vi "Global - UI Stream and Variable Connections.vi"() -> ()   [LabVIEW 2018]
uses:
  support/Message Queue/Message Cluster.ctl
  controls/Variable References.ctl
  controls/Control State.ctl
  controls/IO References.ctl
  support/Message Queue/Message Queue.lvlib
panel:
  in  "IO References":T1
  in  "Variable References":T2
  in  "RT Message Stream":refnum<k21>
  in  "UI Command Stream":refnum<k21>
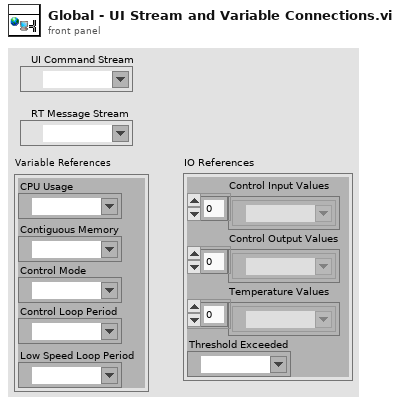
[diagram p1: front panel]
types:
  T1 = typedef "IO References.ctl" = cluster{"Control Input Values":refnum<k21>[], "Control Output Values":refnum<k21>[], "Temperature Values":refnum<k21>[], "Threshold Exceeded":refnum<k21>}
  T2 = typedef "Variable References.ctl" = cluster{"CPU Usage":refnum<k21>, "Contiguous Memory":refnum<k21>, "Control Mode":refnum<k21>, "Control Loop Period":refnum<k21>, "Low Speed Loop Period":refnum<k21>}
diagram:
